vi "RobSteerAdjust.vi"(7 "EncoderTicksPerRev":dbl=1988.0, 9 "Set In":dbl, 11 "Encoder":dbl) -> (3 "Set Out":dbl)   [LabVIEW 2014]
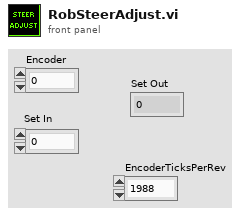
[diagram p1: front panel]
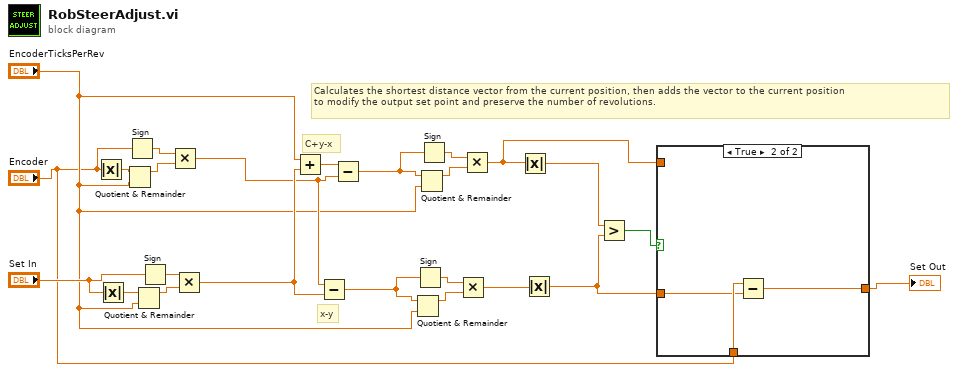
[diagram p0: block diagram]
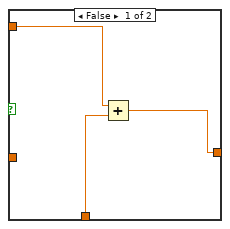
[diagram p2: hidden frame]
diagram:
  # "Calculates the shortest distance vector from the current position, then adds the vector to the current position\nto modify the output set point and preserve the number of revolutions."
  # "x-y"
  # "C+y-x"
  n1 = Absolute Value(x="Encoder") -> (abs(x)=w7:dbl)
  n2 = Absolute Value(x="Set In") -> (abs(x)=w6:dbl)
  n3 = Quotient & Remainder(x=w7, y="EncoderTicksPerRev") -> (x-y*floor(x/y)=w23:dbl)  [unwired: 1 out]
  n4 = Sign(1:"Encoder") -> (0:w24:dbl)
  n5 = Quotient & Remainder(x=w6, y="EncoderTicksPerRev") -> (x-y*floor(x/y)=w22:dbl)  [unwired: 1 out]
  n6 = Sign(1:"Set In") -> (0:w21:dbl)
  n7 = Multiply(x=w24, y=w23) -> (x*y=w9:dbl)
  n8 = Multiply(x=w21, y=w22) -> (x*y=w16:dbl)
  n9 = Add(x="EncoderTicksPerRev", y=w16) -> (x+y=w20:dbl)
  n10 = Subtract(x=w9, y=w16) -> (x-y=w13:dbl)
  n11 = Subtract(x=w20, y=w9) -> (x-y=w17:dbl)
  n12 = Quotient & Remainder(x=w13, y="EncoderTicksPerRev") -> (x-y*floor(x/y)=w14:dbl)  [unwired: 1 out]
  n13 = Sign(1:w13) -> (0:w15:dbl)
  n14 = Quotient & Remainder(x=w17, y="EncoderTicksPerRev") -> (x-y*floor(x/y)=w18:dbl)  [unwired: 1 out]
  n15 = Sign(1:w17) -> (0:w19:dbl)
  n16 = Multiply(x=w15, y=w14) -> (x*y=w10:dbl)
  n17 = Multiply(x=w19, y=w18) -> (x*y=w8:dbl)
  n18 = Absolute Value(x=w8) -> (abs(x)=w12:dbl)
  n19 = Absolute Value(x=w10) -> (abs(x)=w1:dbl)
  n20 = Greater?(x=w12, y=w1) -> (0:w11:bool)
  n21 = case shown="True" w11 {
    tunnel: "Encoder" -> [w26 w29]
    tunnel: [w25 w30] -> w3
    tunnel: w8 -> [w27 _]
    tunnel: w1 -> [_ w28]
    frame False {
      n22 = Add(x=w27, y=w26) -> (x+y=w25:dbl)
    }
    frame True {
      n23 = Subtract(x=w29, y=w28) -> (x-y=w30:dbl)
    }
  }
  "Set Out" <- w3
